vi "Kxx_Kxy_B_cs580.vi"() -> ()   [LabVIEW 2023]
uses:
  <instrlib>/Keithley 622x LV 2009/Keithley 622x.lvlib
  <instrlib>/Keithley 622x LV 2009/Utility/Typedefs/KE622x -- Instrument Type.ctl
  <vilib>/Analysis/NI_AALBase.lvlib
  <instrlib>/Keithley 24XX/Keithley 24XX.lvlib
  <vilib>/Analysis/1siggen.llb/Ramp Pattern by Samples.vi
  Global Variables/MQM Data Transfer All.vi
  <vilib>/Analysis/baseanly.llb/Mean (DBL).vi
  Typedefs/Kxx_Kxy_state_machine_cases.ctl
  Global Variables/Thermometers.vi
  <vilib>/Utility/file.llb/Read Delimited Spreadsheet (DBL).vi
  <vilib>/Instr/_visa.llb/VISA Configure Serial Port (Instr).vi
  <vilib>/Utility/file.llb/Write To Spreadsheet File (string).vi
panel:
  in  "Kxy data":dbl[](array[numeric])
  in  "Kxx data":dbl[](array[numeric])
  in  "T_avg data":dbl[](array[numeric])
  in  "dTxx":dbl
  in  "HTR Power":dbl
  in  "dTxy":dbl
  in  "T_avg":dbl
  in  "T_H Array":dbl[](array[numeric])
  in  "T_C1 Array":dbl[](array[numeric])
  in  "T_C2 Array":dbl[](array[numeric])
  in  "HTR Voltage Array":dbl[](array[numeric])
  in  "?":enum32{"Setup", "Plotting", "Error Readouts"}(tab)
  in  "DeltaT (fraction of tsp)":dbl=0.05
  in  "Sample_t":dbl
  in  "Sample_w":dbl
  in  "Sample_Lxx":dbl
  in  "Heater Current File (H, T, current)":path
  out "Heater Current \nArray":dbl[](array[numeric])
  out "Ramp Pattern":dbl[](array[numeric])
  in  "Tstart (K)":dbl=3.0
  in  "Tend (K)":dbl=4.0
  in  "Steps":i16=2
  in  "Log (on)\nLin (off) (Temperature setpoints)":bool=TRUE
  in  "Initial Heater Current (A)":dbl=1e-06
  in  "Hstart (Oe)":dbl
  in  "Hend (Oe)":dbl
  in  "Field Steps":i16=1
  in  "Log (on)\nLin (off)  (Field setpoints)":bool
  in  "Sample_Lxy":dbl=0.0005
  in  "Test?":bool
  in  "Calibration Only?":bool
  in  "Exchange gas?":bool
  in  "Preset Heater Current Array?":bool
  in  "T Current Source":refnum<visa-resource-name>="6221B"
  in  "HTR Current Source":refnum<visa-resource-name>="CS580-1"
  in  "DC Voltmeter":refnum<visa-resource-name>="2182"
  in  "Thermometer Frequency (Hz)":string="37"
  in  "Initial Thermometer Current (A)":string="1.4142e-7"
  in  "Final Field (Oe)":dbl
  in  "Final Temperature (K)":dbl=1.7
  in  "Filename":path=path "C:/User Data/Luke/Kxx/NaYSe2/NaYSe2_1p7_100K_log_100_9T_8_23_21"
  in  "Heater Only?":bool
  in  "Running avg size":dbl=500.0 format="%#_13g"
  in  "std/mean thresh":dbl=1e-05 format="%#_13g"
  in  "slope/mean thresh":dbl=1e-07 format="%#_13g"
  out "Kxx Plot":cluster{dbl[], dbl[]}(graph)
  out "Kxy Plot":cluster{dbl[], dbl[]}(graph)
  out "All Data":cluster{dbl[], dbl[]}[](graph)
  in  "Finish":bool
  out "Data Rate (ms)":u32
  in  "Delay (ms)":dbl=300.0
  in  "Quick Data Recording":bool=TRUE
  out "Tsp":dbl
  out "HTR_Current":dbl
  out "Mask":dbl
  out "HTR_Voltage":dbl
  out "T_H":dbl
  out "T_C1":dbl
  out "I_therm":dbl
  out "T_C2":dbl
  in  "Display Elements":cluster{"X":bool, "Y":bool, "Name":u16}[](array[cluster]) {"Name" items=["Time (ms)", "Temperature (K)", "Field (T)", "LI_1_X", "LI_1_theta", "LI_3_X", "LI_3_theta", "LI_2_X", "LI_2_theta", "DC_V", "DC_I", "mask", "tsp", "I_therm", "T_H", "T_C1", "T_C2", "Fieldsp"]}
  in  "X-Axis":u16(ring) items=["Linear", "Reciprocal", "Log10"]
  in  "Y-Axis":u16(ring) items=["Linear", "Reciprocal", "Log10"]
  out "Fieldsp":dbl
  out "Global Stop":bool
  out "Thermometers":cluster{"T_H":dbl, "T_C1":dbl, "T_C2":dbl}
  out "QD error out":errorcluster
  out "KE6221 error out":errorcluster
  out "KE2182 error out":errorcluster
  # "TURN ON HIGH VACUUM!"
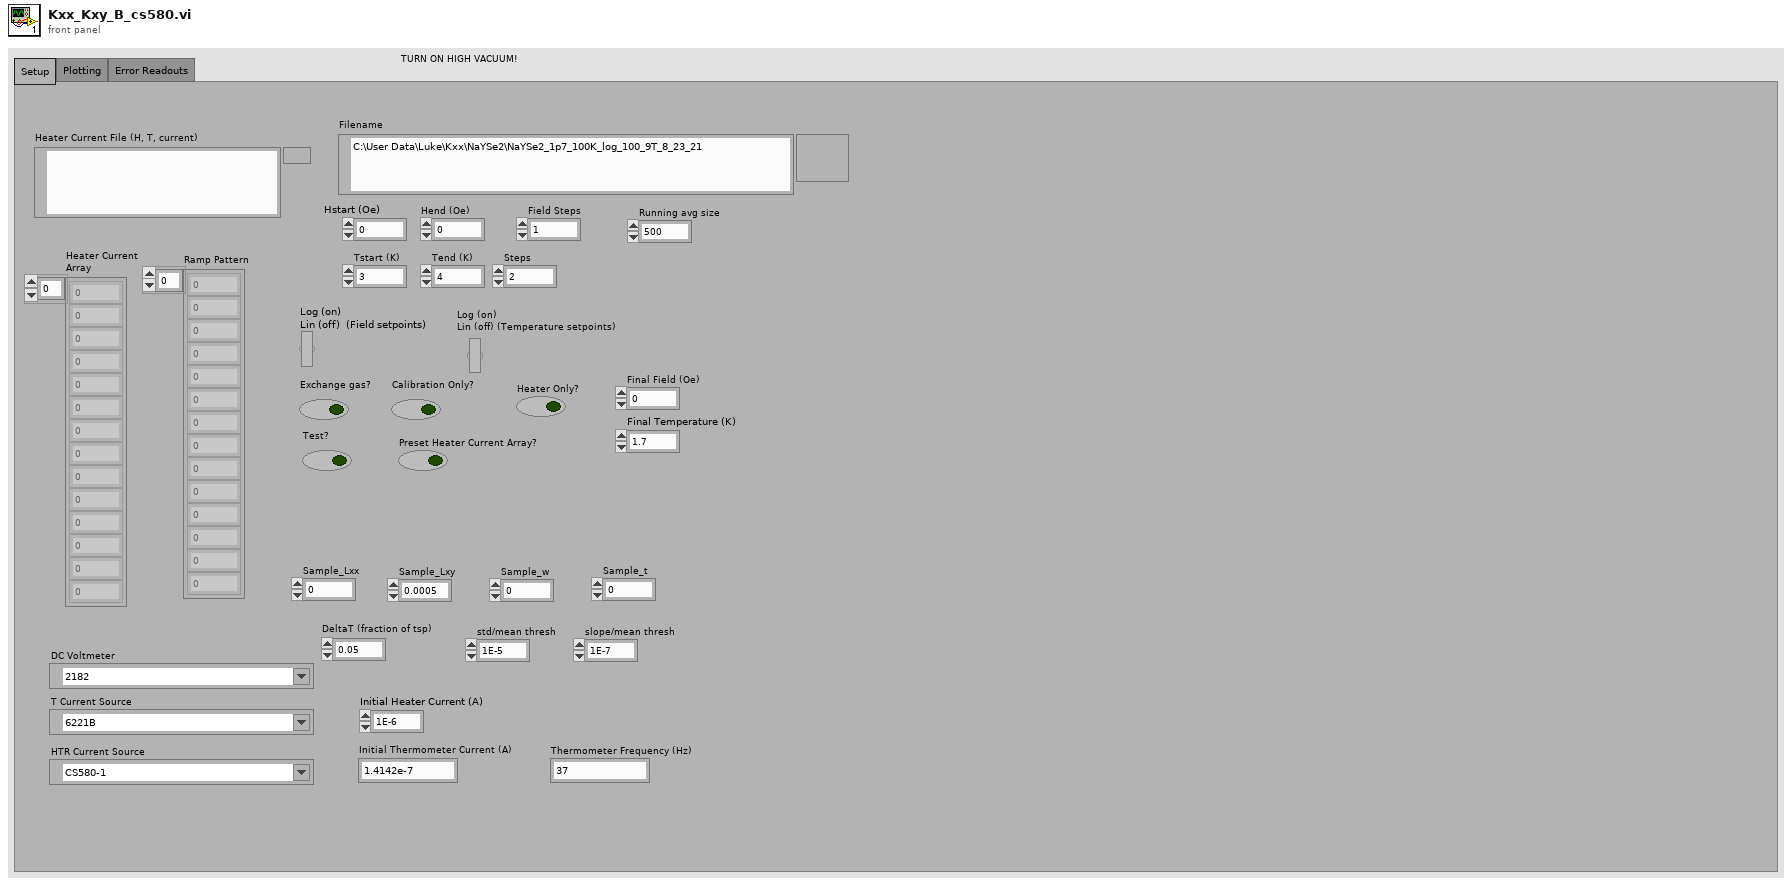
[diagram p1: front panel]
types:
  T1 = typedef "Keithley 622x.lvlib/KE622x -- Instrument Type.ctl" = enum16{"KE6220", "KE6221"}
  T2 = typedef "Kxx_Kxy_state_machine_cases.ctl" = enum16{"Initialize", "Wait to Stabilize (no heat)", "Measure (no heat)", "Turn on Heater, stabilize", "Measure (heat)", "Turn off Heater", "Assign Heater Current", "Plot Kxx, Kxy", "End"}
  T3 = cluster{"T_avg data":dbl[], "Kxx data":dbl[], "Kxy data":dbl[]}
  T4 = cluster{"T_avg":dbl, "dTxx":dbl, "dTxy":dbl, "HTR Power":dbl, "HTR Voltage Array":dbl[], "T_H Array":dbl[], "T_C1 Array":dbl[], "T_C2 Array":dbl[], "error out":errorcluster}
  T5 = typedef "ZI_Frontpanel_All.ctl" = cluster{"Lockin 1 Demod 0":cluster{"R(V)":dbl, "Theta (deg)":dbl, "Timestamp (ms)":u32, "X(V)":dbl, "Y(V)":dbl, "frequency (Hz)":dbl, "output voltage (V)":dbl}, "Lockin 2 Demod 0":cluster{"R(V)":dbl, "Theta (deg)":dbl, "Timestamp (ms)":u32, "X(V)":dbl, "Y(V)":dbl, "frequency (Hz)":dbl, "output voltage (V)":dbl}, "Lockin 3 Demod 0":cluster{"R(V)":dbl, "Theta (deg)":dbl, "Timestamp (ms)":u32, "X(V)":dbl, "Y(V)":dbl, "frequency (Hz)":dbl, "output voltage (V)":dbl}, "Lockin 4 Demod 0":cluster{"R(V)":dbl, "Theta (deg)":dbl, "Timestamp (ms)":u32, "X(V)":dbl, "Y(V)":dbl, "frequency (Hz)":dbl, "output voltage (V)":dbl}, "LI1 active":bool, "LI2 active":bool, "LI3 active":bool, "LI4 active":bool}
  T6 = typedef "PPMS_Status.ctl" = cluster{"Field":cluster{"Field (T)":dbl, "Field stable":bool, "Timestamp (ms)":u32}, "Temperature":cluster{"Temperature (K)":dbl, "Temperature stable":bool, "Timestamp (ms)":u32}}
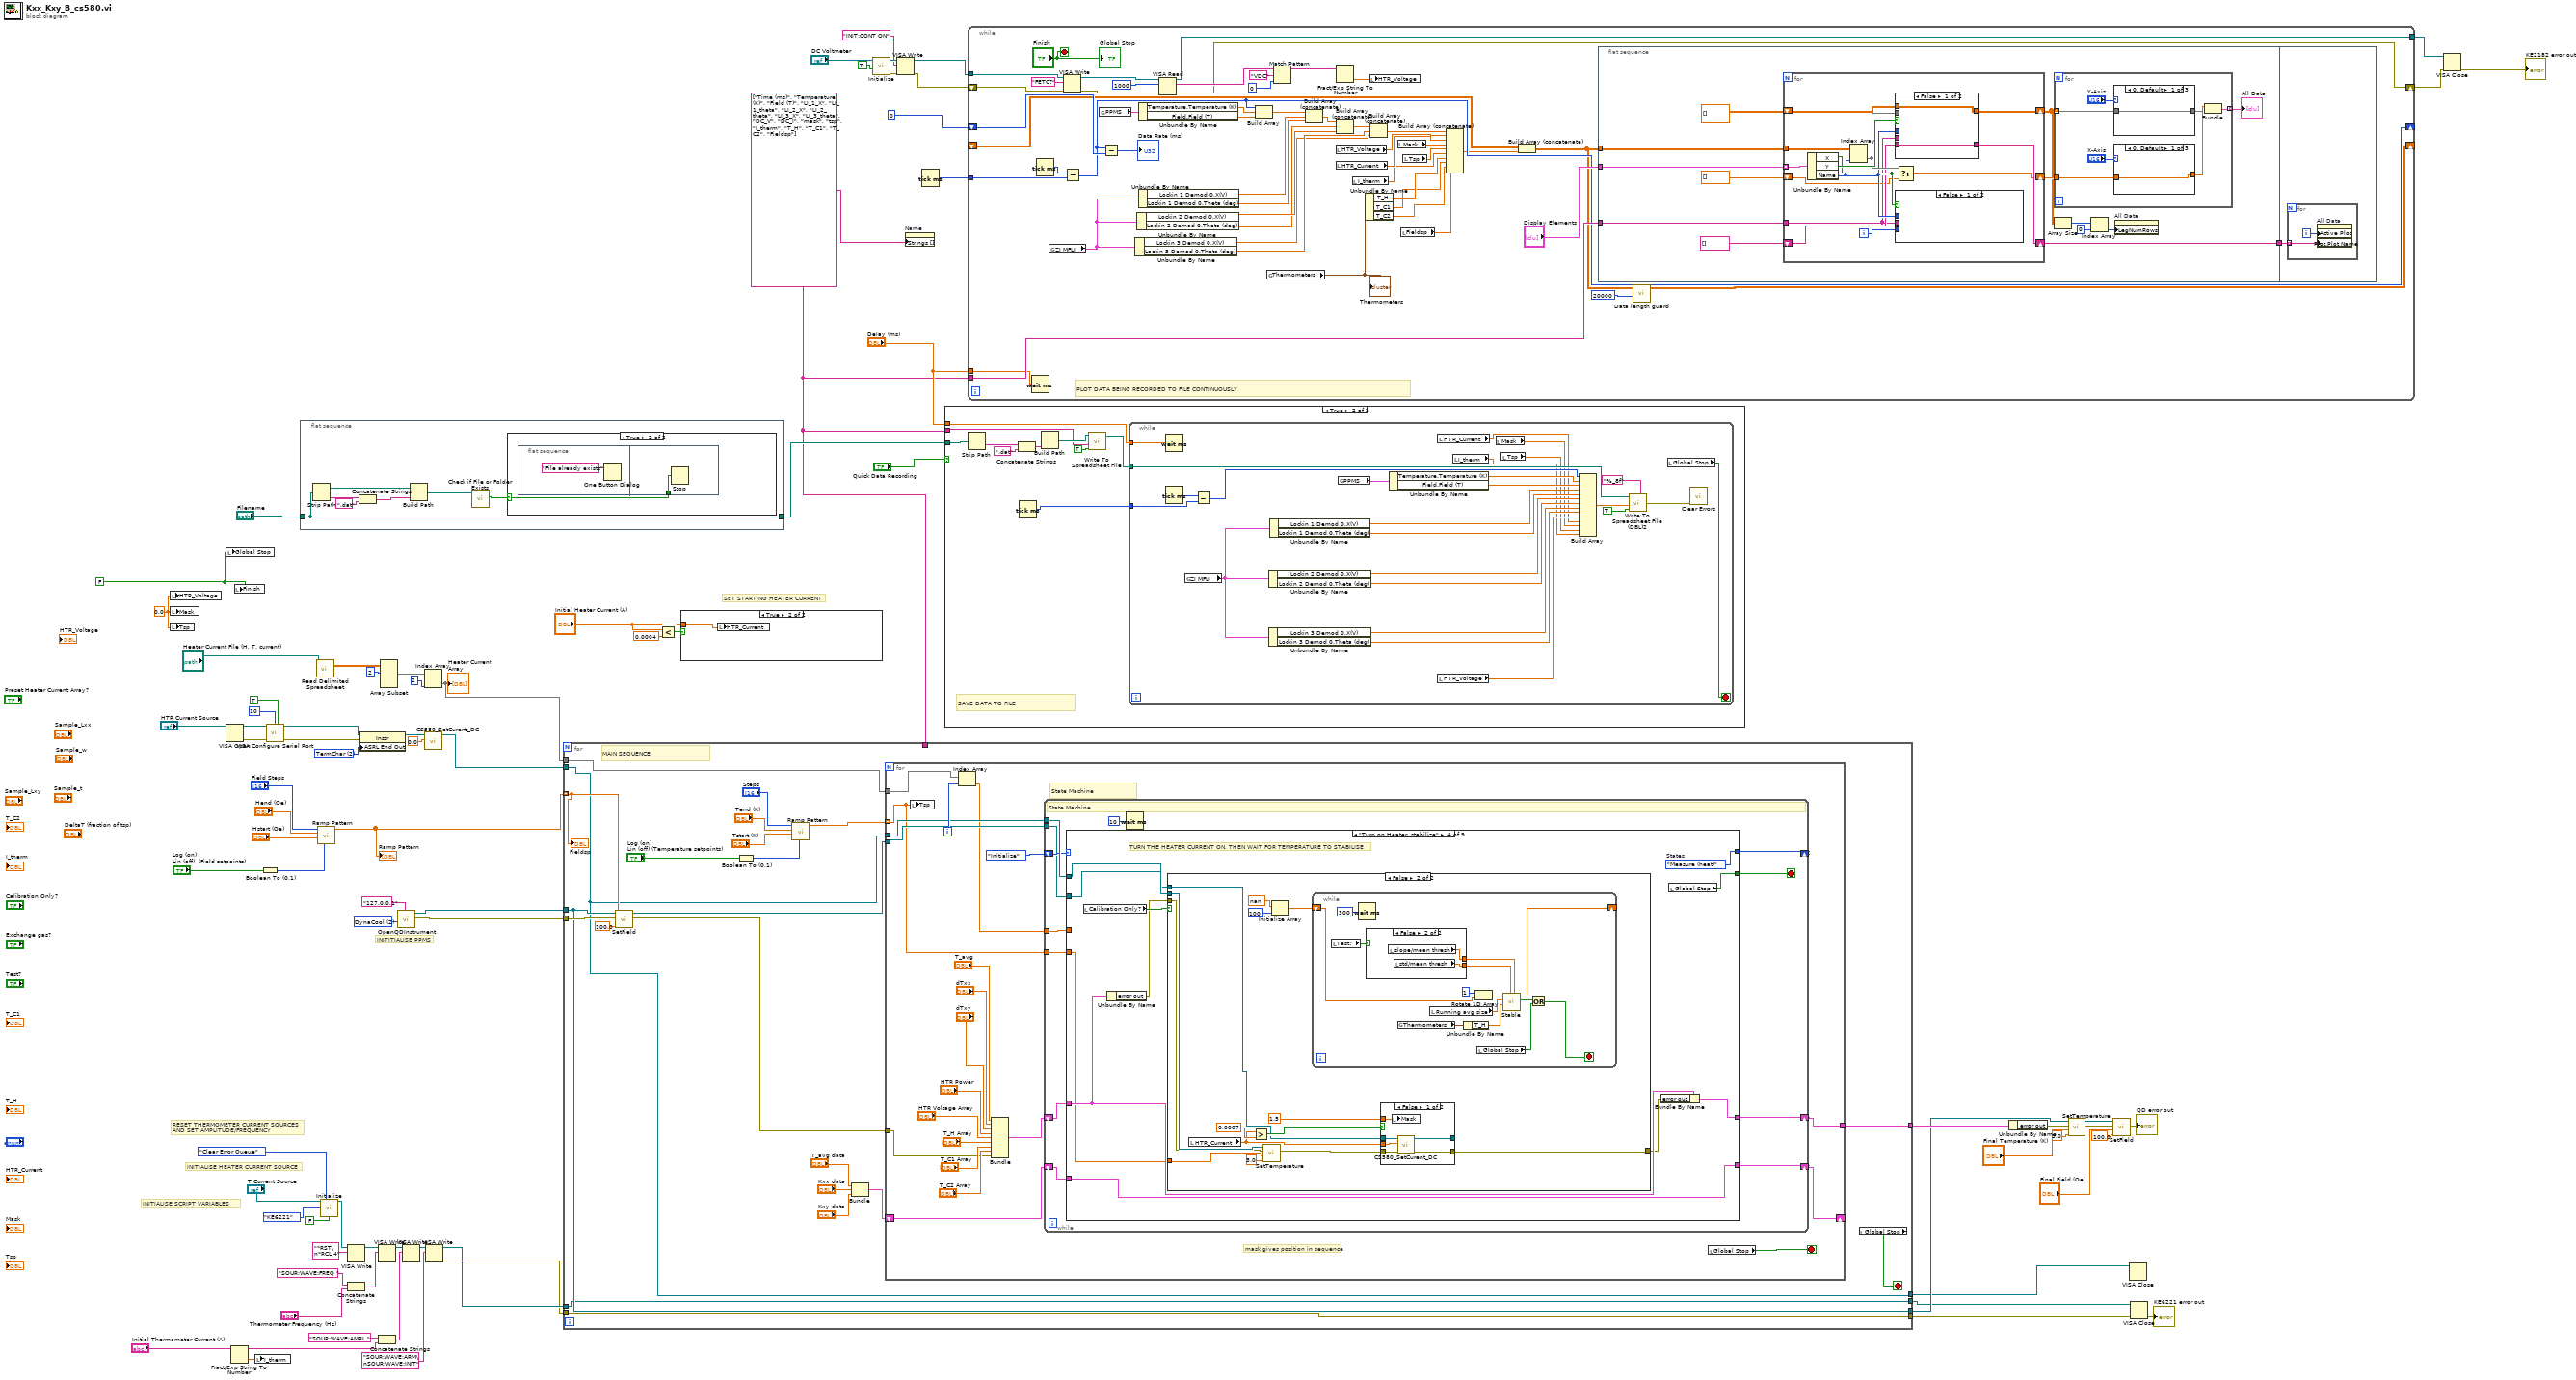
[diagram p0: block diagram]
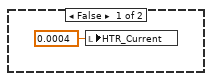
[diagram p2: hidden frame]
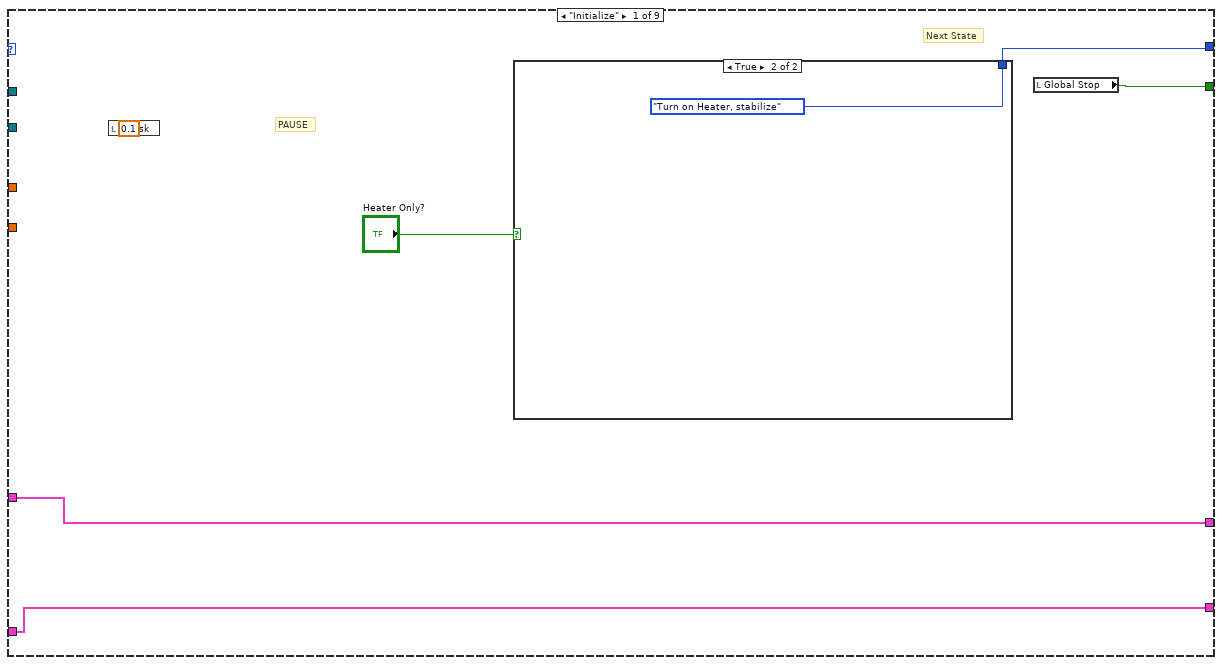
[diagram p4: hidden frame]
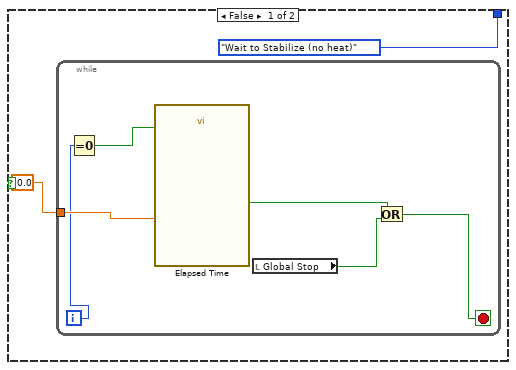
[diagram p5: hidden frame]
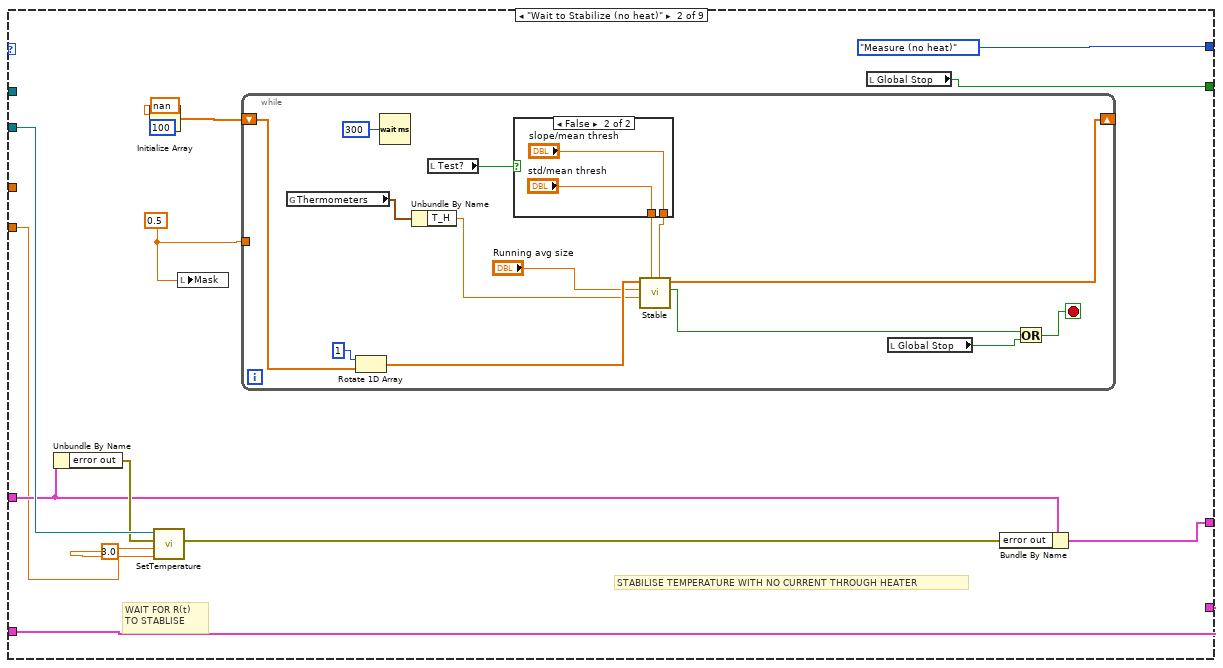
[diagram p6: hidden frame]
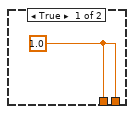
[diagram p7: hidden frame]
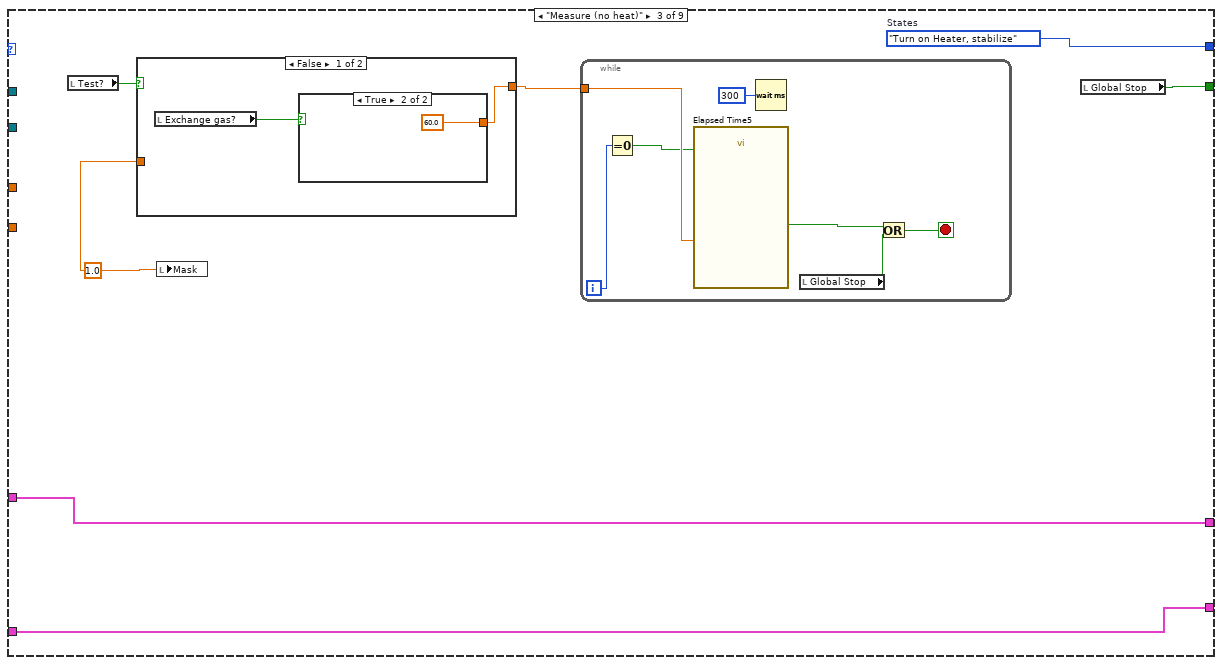
[diagram p8: hidden frame]
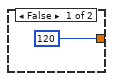
[diagram p9: hidden frame]
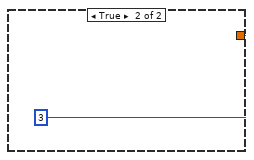
[diagram p10: hidden frame]
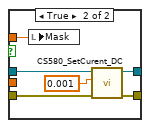
[diagram p12: hidden frame]
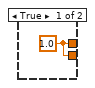
[diagram p13: hidden frame]
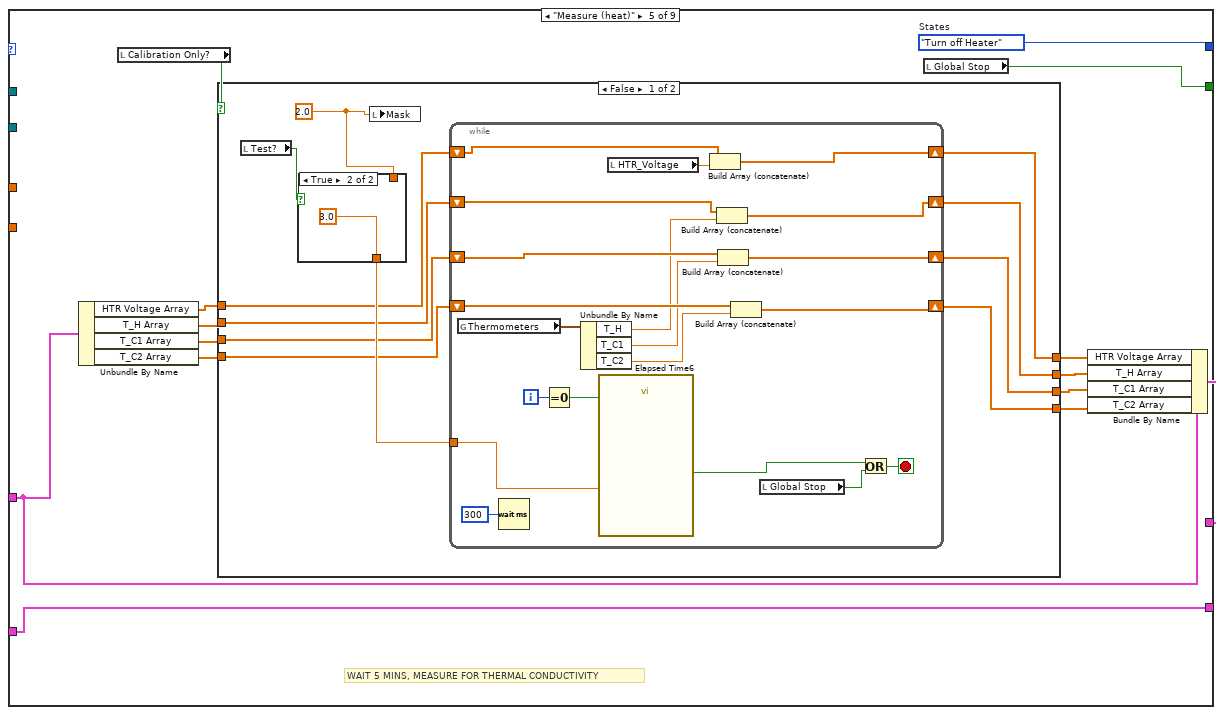
[diagram p14: hidden frame]
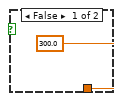
[diagram p15: hidden frame]
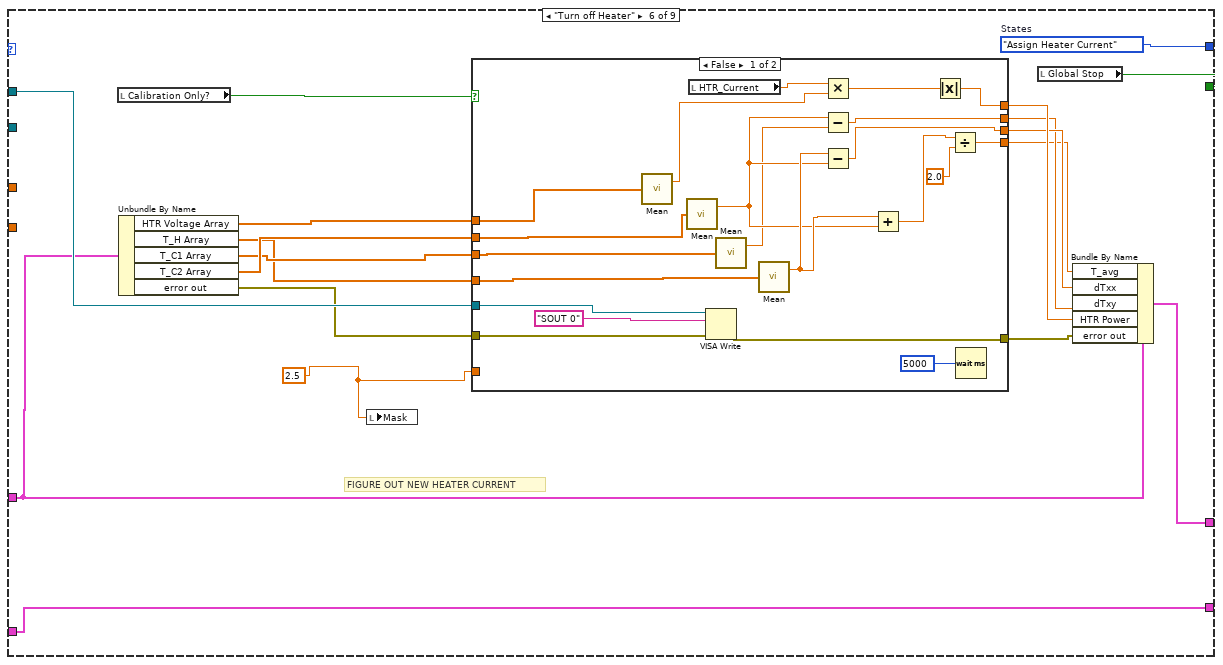
[diagram p17: hidden frame]
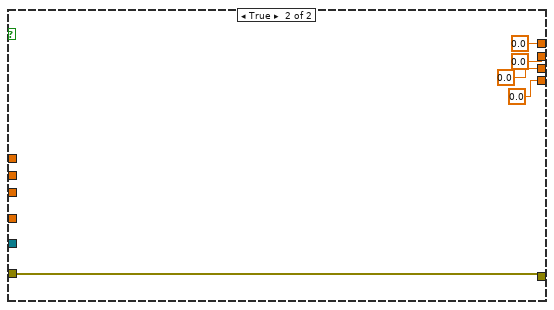
[diagram p18: hidden frame]
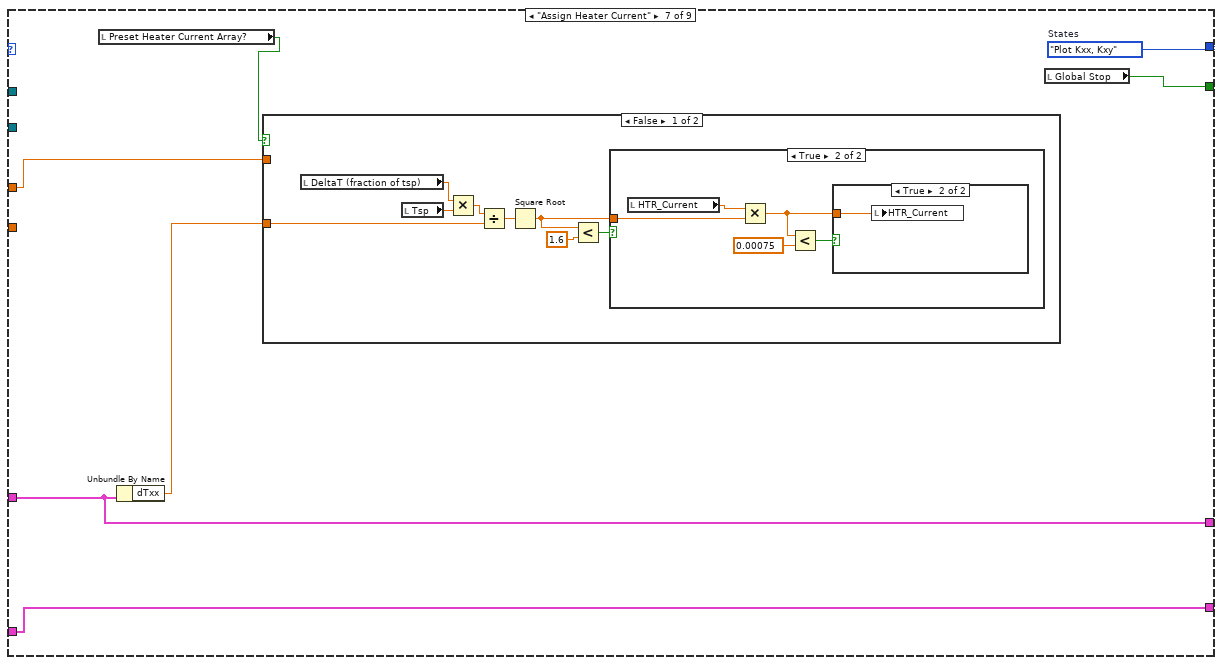
[diagram p19: hidden frame]
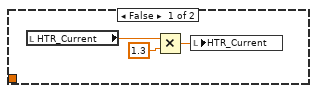
[diagram p20: hidden frame]
diagram:
  w2 = FALSE ("Calibration confirmed")
  w1 = string[] ["Time (ms)", "Temperature (K)", "Field (T)", "LI_1_X", "LI_1_theta", "LI_2_X", "LI_2_theta", "LI_3_X", "LI_3_theta", "DC_V", "DC_I", "mask", "tsp", "I_therm", "T_H", "T_C1", "T_C2", "Fieldsp"] ("element")
  w53 = u16 2 items=["None", "Last Bit", "TermChar", "Break"] ("Serial Settings:End Mode for Writes")
  w71 = 0.0 ("Mask")
  w78 = 2 items=["PPMS", "VersaLab", "DynaCool", "SVSM"] ("Instrument Type")
  # "SET STARTING HEATER CURRENT"
  # "INITIALISE HEATER CURRENT SOURCE"
  # "RESET THERMOMETER CURRENT SOURCES\nAND SET AMPLITUDE/FREQUENCY"
  # "INITITIALISE PPMS"
  # "INITIALISE SCRIPT VARIABLES"
  n1 = local write "HTR_Voltage"(w71) -> ()
  n2 = local write "Mask"(w71) -> ()
  n3 = local write "Tsp"(w71) -> ()
  n4 = VISA Open(VISA resource name="HTR Current Source") -> (VISA resource name=w49:refnum<visa-resource-name>, error out=w50:errorcluster)  [unwired: 4 in]
  n5 = local write "Global Stop"(w2) -> ()
  n6 = Fract/Exp String To Number(string="Initial Thermometer Current (A)") -> (number=w61:dbl)  [unwired: 3 in, 1 out]
  n7 = local write "Finish"(w2) -> ()
  n8 = local write "I_therm"(w61) -> ()
  n9 = Boolean To (0,1)(Boolean="Log (on)\nLin (off)  (Field setpoints)") -> (0, 1=w56:i16)
  n10 = call-poly "VISA Configure Serial Port"("VISA resource name"=w49, "termination char\n(0xA = '\\n' = LF)"=u8 10 ("termination char\n(0xA = '\\n' = LF)"), "Enable Termination\nChar (T)"=TRUE ("Enable Termination\nChar (T)"), "error in (no error)"=w50) -> ("VISA resource name out"=w51:refnum<visa-resource-name>, "error out"=w52:errorcluster)  [unwired: 10 in]
  n11 = flat-sequence {
    tunnel: "Filename" -> [w85]
    tunnel: [w85] -> w22
    frame #0 {
      n12 = Strip Path(path=w85) -> (stripped path=w89:path, name=w86:string)
      n13 = Concatenate Strings(w86, ".dat") -> (w88:string)
      n14 = Build Path(base path=w89, name or relative path=w88) -> (appended path=w84:path)
      n15 = call <vilib>:"Check if File or Folder Exists.vi"("path"=w84) -> ("file or folder exists?"=w83:bool)  [unwired: 8 in, 2 out]
      n16 = case shown="True" w83 {
        selector: w83 -> [_ w90]
        frame False {
        }
        frame True {
          n17 = flat-sequence {
            tunnel: w90 -> [w92]
            frame #0 {
              n18 = One Button Dialog(message="File already exists") -> ()  [unwired: 1 in, 1 out]
            }
            frame #1 {
              n19 = Stop(stop? (T)=w92) -> ()
            }
          }
        }
      }
    }
  }
  n20 = call-poly <vilib>:"Read Delimited Spreadsheet.vi"("file path (dialog if empty)"="Heater Current File (H, T, current)") -> ("all rows"=w44:dbl[][])  [unwired: 9 in, 5 out]
  n21 = call-poly <vilib>:"Ramp Pattern.vi"("type"=w56, "start"="Hstart (Oe)", "end"="Hend (Oe)", "samples"="Field Steps") -> ("Ramp Pattern"=w38:dbl[])  [unwired: 6 in, 1 out]
  "Ramp Pattern" <- w38
  n22 = call <instrlib>:"Initialize.vi"("VISA resource name"="T Current Source", "Error Queue Option"=enum16{"Clear Error Queue", "Error Query"}."Clear Error Queue", "Instrument Type"=KE622x_--_Instrument_Type."KE6221", "Reset? (T)"=FALSE) -> ("VISA resource name out"=w69:refnum<visa-resource-name>)  [unwired: 10 in, 1 out]
  n23 = VISA Write(VISA resource name=w69, write buffer="*RST\n*RCL 4") -> (VISA resource name out=w63:refnum<visa-resource-name>)  [unwired: 1 in, 2 out]
  n24 = Concatenate Strings("SOUR:WAVE:FREQ " ("string"), "Thermometer Frequency (Hz)") -> (w68:string)
  n25 = property class="Instr"(reference=w51, error in=w52, "ASRL End Out"=w53) -> (reference out=w47:refnum<visa-resource-name>)  [unwired: 1 out]
  n26 = VISA Write(VISA resource name=w63, write buffer=w68) -> (VISA resource name out=w62:refnum<visa-resource-name>)  [unwired: 1 in, 2 out]
  n27 = Concatenate Strings("SOUR:WAVE:AMPL " ("string"), "Initial Thermometer Current (A)") -> (w65:string)
  n28 = Array Subset(array=w44, index (row)=2 ("index")) -> (w42:dbl[][])  [unwired: 3 in]
  n29 = call <instrlib>:"OpenQDInstrument.vi"("IP Address"="127.0.0.1", "Instrument Type"=w78) -> ("error out"=w21:errorcluster, "Instrument Ref"=w19:refnum<k24>)  [unwired: 6 in]
  n30 = VISA Write(VISA resource name=w62, write buffer=w65) -> (VISA resource name out=w39:refnum<visa-resource-name>)  [unwired: 1 in, 2 out]
  n31 = Index Array(array=w42, index (col)=2 ("disabled index (col)")) -> (element=w37:dbl[])  [unwired: 1 in]
  "Heater Current \nArray" <- w37
  n32 = call "CS580_SetCurent_DC.vi"("Current (A)"=0.0, "VISA Refnum in"=w47) -> ("VISA resource name out"=w20:refnum<visa-resource-name>)  [unwired: 8 in, 1 out]
  n33 = VISA Write(VISA resource name=w39, write buffer="SOUR:WAVE:ARM\nSOUR:WAVE:INIT") -> (VISA resource name out=w12:refnum<visa-resource-name>, error out=w8:errorcluster)  [unwired: 1 in, 1 out]
  n34 = for {
    tunnel: w38 -> [w114] mode=indexing
    tunnel: w19 -> [w97]
    tunnel: w21 -> [w112]
    tunnel: w37 -> [w105]
    tunnel: w20 -> [w93]
    tunnel: [w98] -> w14
    tunnel: w12 -> [w96]
    tunnel: [w97] -> w11
    tunnel: [w96] -> w10
    tunnel: w8 -> [w95]
    tunnel: [w95] -> w7
    tunnel: [w93] -> w3
    tunnel: w1 -> [_]
    stop <- w94 stop-if-true
    # "MAIN SEQUENCE"
    n35 = call <instrlib>:"SetField.vi"("Rate"=100.0, "Field"=w114, "error in (no error)"=w112, "Instrument Ref In"=w97) -> ("error out"=w104:errorcluster, "Instrument Ref Out"=w103:refnum<k24>)  [unwired: 3 in, 1 out]
    n36 = Boolean To (0,1)(Boolean="Log (on)\nLin (off) (Temperature setpoints)") -> (0, 1=w109:i16)
    n37 = call-poly <vilib>:"Ramp Pattern.vi"("type"=w109, "start"="Tstart (K)", "end"="Tend (K)", "samples"="Steps") -> ("Ramp Pattern"=w111:dbl[])  [unwired: 6 in, 1 out]
    n38 = Bundle("T_avg data"="T_avg data", "Kxx data"="Kxx data", "Kxy data"="Kxy data") -> (w99:T3)  [unwired: 1 in]
    n39 = for {
      tunnel: w111 -> [w117] mode=indexing
      tunnel: w105 -> [w135]
      tunnel: w104 -> [w122]
      tunnel: w93 -> [w132]
      tunnel: w103 -> [w131]
      shift-right: [w116] -> _
      shift-left: w99 -> [w115]
      tunnel: [w119] -> w98
      i -> [w134]
      stop <- w118 stop-if-true
      # "State Machine"
      # "mask gives position in sequence"
      n40 = local write "Tsp"(w117) -> ()
      n41 = Index Array(array=w135, index=w134) -> (element=w120:dbl)
      n42 = Bundle("T_avg"="T_avg", "dTxx"="dTxx", "dTxy"="dTxy", "HTR Power"="HTR Power", "HTR Voltage Array"="HTR Voltage Array", "T_H Array"="T_H Array", "T_C1 Array"="T_C1 Array", "T_C2 Array"="T_C2 Array", "error out"=w122) -> (w121:T4)  [unwired: 1 in]
      n43 = while {
        shift-right: [w147] -> _
        shift-left: Kxx_Kxy_state_machine_cases."Initialize" -> [w144]
        tunnel: w132 -> [w145]
        tunnel: w131 -> [w140]
        shift-right: [w143] -> w119
        shift-left: w121 -> [w142]
        tunnel: w120 -> [w141]
        tunnel: w117 -> [w138]
        shift-right: [w137] -> w116
        shift-left: w115 -> [w136]
        stop <- w139 stop-if-true
        # "State Machine"
        n44 = case shown="\"Turn on Heater, stabilize\"" w144 {
          selector: w144 -> [_ _ _ _ _ _ _ _ w418]
          tunnel: w140 -> [_ w172 _ w222 _ _ _ _ _]
          tunnel: [w152 Kxx_Kxy_state_machine_cases."Measure (no heat)" w198 w220 w280 w334 w368 w406 w418] -> w147
          tunnel: w145 -> [_ _ _ w221 _ w335 _ _ _]
          tunnel: [w151 w168 w197 w216 w271 w322 w366 w405 w417] -> w143
          tunnel: w142 -> [w151 w169 w197 w218 w270 w329 w366 w405 w417]
          tunnel: w136 -> [w150 w167 w196 w215 w269 w321 w365 w396 w416]
          tunnel: [w150 w167 w196 w215 w269 w321 w365 w392 w416] -> w137
          tunnel: w141 -> [_ _ _ _ _ _ w364 _ _]
          tunnel: [w149 w166 w195 w214 w268 w320 w363 w389 TRUE] -> w139
          tunnel: w138 -> [_ w165 _ w213 _ _ _ _ _]
          frame "Initialize" {
            # "Next State"
            # "PAUSE"
            n45 = local write "Mask"(0.1 ("Mask")) -> ()
            n46 = case shown="True" "Heater Only?" {
              tunnel: [Kxx_Kxy_state_machine_cases."Wait to Stabilize (no heat)" Kxx_Kxy_state_machine_cases."Turn on Heater, stabilize"] -> w152
              frame False {
                n47 = while {
                  tunnel: 10.0 ("Time Target (s)") -> [w161]
                  i -> [w157]
                  stop <- w158 stop-if-true
                  n48 = Equal To 0?(x=w157) -> (x = 0?=w156:bool)
                  n49 = call "Elapsed Time"("Time Target (s)"=w161, "Reset"=w156) -> ("Time has Elapsed"=w160:bool)  [unwired: 10 in, 7 out]
                  n50 = local read "Global Stop"() -> (w159:bool)
                  n51 = Or(x=w160, y=w159) -> (x .or. y?=w158:bool)
                }
              }
              frame True {
              }
            }
            n52 = local read "Global Stop"() -> (w149:bool)
          }
          frame "Wait to Stabilize (no heat)" {
            w163 = 0.5 ("Mask")
            # "STABILISE TEMPERATURE WITH NO CURRENT THROUGH HEATER"
            # "WAIT FOR R(t)\nTO STABLISE"
            n53 = Unbundle By Name(w169) -> ("error out"=w170:errorcluster)
            n54 = Initialize Array(nan ("Element"), 100) -> (w176:dbl[])
            n55 = call <instrlib>:"SetTemperature.vi"("Rate"=3.0, "Temperature"=w165, "error in (no error)"=w170, "Instrument Ref In"=w172) -> ("error out"=w164:errorcluster)  [unwired: 3 in, 2 out]
            n56 = local write "Mask"(w163) -> ()
            n57 = while {
              shift-right: [w179] -> _
              shift-left: w176 -> [w189]
              tunnel: w163 -> [_]
              stop <- w185 stop-if-true
              n58 = global read "Thermometers.vi" "Thermometers"() -> (w184:cluster{"T_H":dbl, "T_C1":dbl, "T_C2":dbl})
              n59 = Rotate 1D Array(1:w189, 2:1 ("n")) -> (0:w183:dbl[])
              n60 = Wait (ms)(milliseconds to wait=u32 300) -> ()  [unwired: 1 out]
              n61 = Unbundle By Name(w184) -> ("T_H"=w181:dbl)
              n62 = local read "Test?"() -> (w187:bool)
              n63 = case shown="False" w187 {
                tunnel: [w191 "slope/mean thresh"] -> w180
                tunnel: [w191 "std/mean thresh"] -> w177
                frame True {
                  w191 = 1.0 ("y")
                }
                frame False {
                }
              }
              n64 = call "Stable.vi"("slope/mean thresh"=w180, "std/mean thresh"=w177, "New data point"=w181, "Number of points"="Running avg size", "Array in"=w183) -> ("Stable?"=w178:bool, "Array out"=w179:dbl[])  [unwired: 5 in]
              n65 = local read "Global Stop"() -> (w186:bool)
              n66 = Or(x=w178, y=w186) -> (x .or. y?=w185:bool)
            }
            n67 = local read "Global Stop"() -> (w166:bool)
            n68 = Bundle By Name(cluster=w169, "error out"=w164) -> (w168:T4)
          }
          frame "Measure (no heat)" {
            w198 = Kxx_Kxy_state_machine_cases."Turn on Heater, stabilize"  # States
            w194 = 1.0 ("Mask")
            n69 = local read "Test?"() -> (w200:bool)
            n70 = case shown="False" w200 {
              tunnel: [w201 u32 3 ("milliseconds to wait")] -> w199
              tunnel: w194 -> [_ _]
              frame False {
                n71 = local read "Exchange gas?"() -> (w202:bool)
                n72 = case shown="True" w202 {
                  tunnel: [120 60.0 ("Time to Wait (s)")] -> w201
                  frame False {
                  }
                  frame True {
                  }
                }
              }
              frame True {
              }
            }
            n73 = local write "Mask"(w194) -> ()
            n74 = while {
              tunnel: w199 -> [w210]
              i -> [w207]
              stop <- w209 stop-if-true
              n75 = Equal To 0?(x=w207) -> (x = 0?=w206:bool)
              n76 = call "Elapsed Time5"("Time Target (s)"=w210, "Reset"=w206) -> ("Time has Elapsed"=w208:bool)  [unwired: 10 in, 7 out]
              n77 = Wait (ms)(milliseconds to wait=u32 300) -> ()  [unwired: 1 out]
              n78 = local read "Global Stop"() -> (w212:bool)
              n79 = Or(x=w208, y=w212) -> (x .or. y?=w209:bool)
            }
            n80 = local read "Global Stop"() -> (w195:bool)
          }
          frame "Turn on Heater, stabilize" {
            w220 = Kxx_Kxy_state_machine_cases."Measure (heat)"  # States
            # "TURN THE HEATER CURRENT ON, THEN WAIT FOR TEMPERATURE TO STABILISE"
            n81 = local read "Calibration Only?"() -> (w223:bool)
            n82 = Unbundle By Name(w218) -> ("error out"=w219:errorcluster)
            n83 = case shown="False" w223 {
              tunnel: w222 -> [_ w238]
              tunnel: w219 -> [w224 w230]
              tunnel: [w224 w231] -> w217
              tunnel: w221 -> [_ w232]
              tunnel: w213 -> [_ w227]
              frame True {
              }
              frame False {
                n84 = local read "HTR_Current"() -> (w225:dbl)
                n85 = Greater?(x=w225, y=0.0007) -> (0:w233:bool)
                n86 = call <instrlib>:"SetTemperature.vi"("Rate"=3.0, "Temperature"=w227, "error in (no error)"=w230, "Instrument Ref In"=w238) -> ("error out"=w229:errorcluster)  [unwired: 3 in, 2 out]
                n87 = Initialize Array(nan ("Element"), 100) -> (w237:dbl[])
                n88 = while {
                  shift-right: [w261] -> _
                  shift-left: w237 -> [w263]
                  stop <- w259 stop-if-true
                  n89 = local read "Test?"() -> (w260:bool)
                  n90 = Wait (ms)(milliseconds to wait=u32 300) -> ()  [unwired: 1 out]
                  n91 = case shown="False" w260 {
                    tunnel: [w265 w267] -> w253
                    tunnel: [w265 w266] -> w252
                    frame True {
                      w265 = 1.0 ("y")
                    }
                    frame False {
                      n92 = local read "slope/mean thresh"() -> (w267:dbl)
                      n93 = local read "std/mean thresh"() -> (w266:dbl)
                    }
                  }
                  n94 = global read "Thermometers.vi" "Thermometers"() -> (w257:cluster{"T_H":dbl, "T_C1":dbl, "T_C2":dbl})
                  n95 = local read "Running avg size"() -> (w251:dbl)
                  n96 = Unbundle By Name(w257) -> ("T_H"=w254:dbl)
                  n97 = Rotate 1D Array(1:w263, 2:1 ("n")) -> (0:w255:dbl[])
                  n98 = local read "Global Stop"() -> (w258:bool)
                  n99 = call "Stable.vi"("slope/mean thresh"=w253, "std/mean thresh"=w252, "New data point"=w254, "Number of points"=w251, "Array in"=w255) -> ("Stable?"=w256:bool, "Array out"=w261:dbl[])  [unwired: 5 in]
                  n100 = Or(x=w256, y=w258) -> (x .or. y?=w259:bool)
                }
                n101 = case shown="False" w233 {
                  tunnel: w229 -> [w242 w250]
                  tunnel: w232 -> [w243 w249]
                  tunnel: [w240 w248] -> w231
                  tunnel: [w241 w247] -> _
                  tunnel: w225 -> [w244 _]
                  tunnel: 1.5 ("Mask") -> [w239 w245]
                  frame False {
                    n102 = local write "Mask"(w239) -> ()
                    n103 = call "CS580_SetCurent_DC.vi"("error in"=w242, "Current (A)"=w244, "VISA Refnum in"=w243) -> ("error out"=w240:errorcluster, "VISA resource name out"=w241:refnum<visa-resource-name>)  [unwired: 7 in]
                  }
                  frame True {
                    n104 = local write "Mask"(w245) -> ()
                    n105 = call "CS580_SetCurent_DC.vi"("error in"=w250, "Current (A)"=0.001, "VISA Refnum in"=w249) -> ("error out"=w248:errorcluster, "VISA resource name out"=w247:refnum<visa-resource-name>)  [unwired: 7 in]
                  }
                }
              }
            }
            n106 = Bundle By Name(cluster=w218, "error out"=w217) -> (w216:T4)
            n107 = local read "Global Stop"() -> (w214:bool)
          }
          frame "Measure (heat)" {
            w280 = Kxx_Kxy_state_machine_cases."Turn off Heater"  # States
            # "WAIT 5 MINS, MEASURE FOR THERMAL CONDUCTIVITY"
            n108 = Unbundle By Name(w270) -> ("HTR Voltage Array"=w279:dbl[], "T_H Array"=w278:dbl[], "T_C1 Array"=w277:dbl[], "T_C2 Array"=w276:dbl[])
            n109 = local read "Calibration Only?"() -> (w281:bool)
            n110 = case shown="False" w281 {
              tunnel: w279 -> [w290 w318]
              tunnel: w278 -> [w287 w317]
              tunnel: w277 -> [w286 w316]
              tunnel: w276 -> [w285 w315]
              tunnel: [w289 w318] -> w275
              tunnel: [w284 w317] -> w274
              tunnel: [w283 w316] -> w273
              tunnel: [w282 w315] -> w272
              frame False {
                w288 = 2.0 ("Mask")
                n111 = local read "Test?"() -> (w292:bool)
                n112 = case shown="True" w292 {
                  tunnel: [300.0 3.0] -> w291
                  tunnel: w288 -> [_ _]
                  frame False {
                  }
                  frame True {
                  }
                }
                n113 = local write "Mask"(w288) -> ()
                n114 = while {
                  shift-right: [w313] -> w284
                  shift-left: w287 -> [w314]
                  shift-right: [w311] -> w282
                  shift-left: w285 -> [w312]
                  shift-right: [w309] -> w289
                  shift-left: w290 -> [w310]
                  shift-right: [w303] -> w283
                  shift-left: w286 -> [w304]
                  tunnel: w291 -> [w299]
                  i -> [w306]
                  stop <- w300 stop-if-true
                  n115 = global read "Thermometers.vi" "Thermometers"() -> (w298:cluster{"T_H":dbl, "T_C1":dbl, "T_C2":dbl})
                  n116 = Wait (ms)(milliseconds to wait=u32 300) -> ()  [unwired: 1 out]
                  n117 = Equal To 0?(x=w306) -> (x = 0?=w305:bool)
                  n118 = Unbundle By Name(w298) -> ("T_H"=w297:dbl, "T_C1"=w296:dbl, "T_C2"=w295:dbl)
                  n119 = call "Elapsed Time6"("Time Target (s)"=w299, "Reset"=w305) -> ("Time has Elapsed"=w302:bool)  [unwired: 10 in, 7 out]
                  n120 = local read "HTR_Voltage"() -> (w308:dbl)
                  n121 = Build Array (concatenate)(w310, w308) -> (w309:dbl[])
                  n122 = Build Array (concatenate)(w314, w297) -> (w313:dbl[])
                  n123 = Build Array (concatenate)(w304, w296) -> (w303:dbl[])
                  n124 = Build Array (concatenate)(w312, w295) -> (w311:dbl[])
                  n125 = local read "Global Stop"() -> (w301:bool)
                  n126 = Or(x=w302, y=w301) -> (x .or. y?=w300:bool)
                }
              }
              frame True {
              }
            }
            n127 = local read "Global Stop"() -> (w268:bool)
            n128 = Bundle By Name(cluster=w270, "HTR Voltage Array"=w275, "T_H Array"=w274, "T_C1 Array"=w273, "T_C2 Array"=w272) -> (w271:T4)
          }
          frame "Turn off Heater" {
            w319 = 2.5 ("Mask")
            w334 = Kxx_Kxy_state_machine_cases."Assign Heater Current"  # States
            # "FIGURE OUT NEW HEATER CURRENT"
            n129 = local read "Calibration Only?"() -> (w336:bool)
            n130 = Unbundle By Name(w329) -> ("HTR Voltage Array"=w333:dbl[], "T_H Array"=w330:dbl[], "T_C1 Array"=w331:dbl[], "T_C2 Array"=w332:dbl[], "error out"=w328:errorcluster)
            n131 = local write "Mask"(w319) -> ()
            n132 = case shown="False" w336 {
              tunnel: w335 -> [w349 _]
              tunnel: w328 -> [w348 w362]
              tunnel: w332 -> [w338 _]
              tunnel: w330 -> [w339 _]
              tunnel: w333 -> [w340 _]
              tunnel: [w356 0.0] -> w325
              tunnel: [w341 0.0] -> w326
              tunnel: [w350 0.0] -> w323
              tunnel: [w347 w362] -> w327
              tunnel: w331 -> [w337 _]
              tunnel: [w343 0.0] -> w324
              tunnel: w319 -> [_ _]
              frame False {
                n133 = call-poly <vilib>:"Mean.vi"("X"=w340) -> ("mean"=w354:dbl)  [unwired: 1 out]
                n134 = call-poly <vilib>:"Mean.vi"("X"=w338) -> ("mean"=w345:dbl)  [unwired: 1 out]
                n135 = local read "HTR_Current"() -> (w355:dbl)
                n136 = VISA Write(VISA resource name=w349, write buffer="SOUT 0", error in (no error)=w348) -> (error out=w347:errorcluster)  [unwired: 2 out]
                n137 = call-poly <vilib>:"Mean.vi"("X"=w337) -> ("mean"=w344:dbl)  [unwired: 1 out]
                n138 = call-poly <vilib>:"Mean.vi"("X"=w339) -> ("mean"=w353:dbl)  [unwired: 1 out]
                n139 = Multiply(x=w355, y=w354) -> (x*y=w342:dbl)
                n140 = Subtract(x=w345, y=w344) -> (x-y=w343:dbl)
                n141 = Subtract(x=w353, y=w345) -> (x-y=w356:dbl)
                n142 = Add(x=w353, y=w345) -> (x+y=w352:dbl)
                n143 = Absolute Value(x=w342) -> (abs(x)=w341:dbl)
                n144 = Divide(x=w352, y=2.0) -> (x/y=w350:dbl)
                n145 = Wait (ms)(milliseconds to wait=u32 5000) -> ()  [unwired: 1 out]
              }
              frame True {
              }
            }
            n146 = local read "Global Stop"() -> (w320:bool)
            n147 = Bundle By Name(cluster=w329, "T_avg"=w323, "dTxx"=w325, "dTxy"=w324, "HTR Power"=w326, "error out"=w327) -> (w322:T4)
          }
          frame "Assign Heater Current" {
            w368 = Kxx_Kxy_state_machine_cases."Plot Kxx, Kxy"  # States
            n148 = local read "Preset Heater Current Array?"() -> (w369:bool)
            n149 = Unbundle By Name(w366) -> ("dTxx"=w367:dbl)
            n150 = case shown="False" w369 {
              tunnel: w367 -> [w375 _]
              tunnel: w364 -> [_ w388]
              frame False {
                n151 = local read "DeltaT (fraction of tsp)"() -> (w370:dbl)
                n152 = local read "Tsp"() -> (w377:dbl)
                n153 = Multiply(x=w370, y=w377) -> (x*y=w376:dbl)
                n154 = Divide(x=w376, y=w375) -> (x/y=w374:dbl)
                n155 = Square Root(x=w374) -> (sqrt(x)=w373:dbl)
                n156 = Less?(x=w373, y=1.6) -> (x < y?=w371:bool)
                n157 = case shown="True" w371 {
                  tunnel: w373 -> [_ w385]
                  frame False {
                    n158 = local read "HTR_Current"() -> (w379:dbl)
                    n159 = Multiply(x=w379, y=1.3) -> (x*y=w378:dbl)
                    n160 = local write "HTR_Current"(w378) -> ()
                  }
                  frame True {
                    n161 = local read "HTR_Current"() -> (w384:dbl)
                    n162 = Multiply(x=w384, y=w385) -> (x*y=w382:dbl)
                    n163 = Less?(x=w382, y=0.00075) -> (x < y?=w381:bool)
                    n164 = case shown="True" w381 {
                      tunnel: w382 -> [_ w387]
                      frame False {
                        n165 = local write "HTR_Current"(0.00075 ("HTR_Current")) -> ()
                      }
                      frame True {
                        n166 = local write "HTR_Current"(w387) -> ()
                      }
                    }
                  }
                }
              }
              frame True {
                n167 = local write "HTR_Current"(w388) -> ()
              }
            }
            n168 = local read "Global Stop"() -> (w363:bool)
          }
          frame "Plot Kxx, Kxy" {
            w406 = Kxx_Kxy_state_machine_cases."End"  # States
            n169 = local read "Sample_Lxx"() -> (w400:dbl)
            n170 = local read "Sample_w"() -> (w402:dbl)
            n171 = local read "Sample_t"() -> (w401:dbl)
            n172 = local read "Sample_Lxy"() -> (w411:dbl)
            n173 = Unbundle By Name(w405) -> ("T_avg"=w404:dbl, "dTxx"=w403:dbl, "dTxy"=w391:dbl, "HTR Power"=w390:dbl)
            n174 = call "Kxx_Kxy_calc.vi"("Sample_w"=w402, "HTR Power"=w390, "Sample_t"=w401, "dTxy"=w391, "dTxx"=w403, "Sample_Lxx"=w400, "Sample_Lxy"=w411) -> ("Kxx"=w410:dbl, "Kxy"=w409:dbl)  [unwired: 3 in]
            n175 = Unbundle By Name(w396) -> ("T_avg data"=w399:dbl[], "Kxx data"=w398:dbl[], "Kxy data"=w397:dbl[])
            n176 = Build Array (concatenate)(w398, w410) -> (w394:dbl[])
            n177 = Build Array (concatenate)(w397, w409) -> (w393:dbl[])
            n178 = Build Array (concatenate)(w399, w404) -> (w395:dbl[])
            n179 = local read "Calibration Only?"() -> (w407:bool)
            n180 = Bundle(w395, w393) -> (w408:cluster{dbl[], dbl[]})  [unwired: 1 in]
            n181 = Bundle(w395, w394) -> (w412:cluster{dbl[], dbl[]})  [unwired: 1 in]
            n182 = Bundle By Name(cluster=w396, "T_avg data"=w395, "Kxx data"=w394, "Kxy data"=w393) -> (w392:T3)
            n183 = case shown="True" w407 {
              tunnel: w412 -> [_ w414]
              tunnel: w408 -> [_ w413]
              frame True {
              }
              frame False {
                "Kxx Plot" <- w414
                "Kxy Plot" <- w413
              }
            }
            n184 = local read "Global Stop"() -> (w389:bool)
          }
          frame "End" {
          }
        }
        n185 = Wait (ms)(milliseconds to wait=u32 10) -> ()  [unwired: 1 out]
      }
      n186 = local read "Global Stop"() -> (w118:bool)
    }
    n187 = local read "Global Stop"() -> (w94:bool)
    "Fieldsp" <- w114
  }
  n188 = Less?(x="Initial Heater Current (A)", y=0.0004) -> (x < y?=w18:bool)
  n189 = case shown="True" w18 {
    tunnel: "Initial Heater Current (A)" -> [_ w420]
    frame False {
      n190 = local write "HTR_Current"(0.0004 ("HTR_Current")) -> ()
    }
    frame True {
      n191 = local write "HTR_Current"(w420) -> ()
    }
  }
  n192 = call <instrlib>:"Initialize.vi"("Reset (True)"=TRUE, "VISA resource name"="DC Voltmeter") -> ("error out"=w74:errorcluster, "VISA resource name out"=w73:refnum<visa-resource-name>)  [unwired: 8 in]
  n193 = VISA Write(VISA resource name=w73, write buffer="INIT:CONT ON", error in (no error)=w74) -> (VISA resource name out=w32:refnum<visa-resource-name>, error out=w31:errorcluster)  [unwired: 1 out]
  n194 = property on="Name" class="Ring (strict)"("Strings []"=w1) -> ()  [unwired: 2 in, 2 out]
  n195 = Tick Count (ms)() -> (millisecond timer value=w23:u32)
  n196 = case shown="True" "Quick Data Recording" {
    tunnel: w22 -> [_ w424]
    tunnel: "Delay (ms)" -> [_ w422]
    tunnel: w1 -> [_ w421]
    frame False {
    }
    frame True {
      # "SAVE DATA TO FILE"
      n197 = Strip Path(path=w424) -> (stripped path=w428:path, name=w425:string)
      n198 = Concatenate Strings(w425, ".dat") -> (w427:string)
      n199 = Tick Count (ms)() -> (millisecond timer value=w431:u32)
      n200 = Build Path(base path=w428, name or relative path=w427) -> (appended path=w429:path)
      n201 = call-poly <vilib>:"Write To Spreadsheet File.vi"("append to file? (new file:F)"=TRUE, "1D data"=w421, "file path (dialog if empty)"=w429) -> ("new file path (Not A Path if cancelled)"=w423:path)  [unwired: 5 in]
      n202 = while {
        tunnel: w431 -> [w456]
        tunnel: w423 -> [w448]
        tunnel: w422 -> [w447]
        stop <- w432 stop-if-true
        n203 = Wait (ms)(milliseconds to wait=w447) -> ()  [unwired: 1 out]
        n204 = Tick Count (ms)() -> (millisecond timer value=w455:u32)
        n205 = global read "MQM Data Transfer All.vi" "ZI MFLI"() -> (w434:T5)
        n206 = Subtract(x=w455, y=w456) -> (x-y=w454:u32)
        n207 = Unbundle By Name(w434) -> ("Lockin 2 Demod 0.X(V)"=w443:dbl, "Lockin 2 Demod 0.Theta (deg)"=w442:dbl)
        n208 = Unbundle By Name(w434) -> ("Lockin 3 Demod 0.X(V)"=w441:dbl, "Lockin 3 Demod 0.Theta (deg)"=w440:dbl)
        n209 = Unbundle By Name(w434) -> ("Lockin 1 Demod 0.X(V)"=w445:dbl, "Lockin 1 Demod 0.Theta (deg)"=w444:dbl)
        n210 = global read "MQM Data Transfer All.vi" "PPMS"() -> (w433:T6)
        n211 = Unbundle By Name(w433) -> ("Temperature.Temperature (K)"=w453:dbl, "Field.Field (T)"=w452:dbl)
        n212 = local read "HTR_Current"() -> (w438:dbl)
        n213 = local read "HTR_Voltage"() -> (w439:dbl)
        n214 = local read "I_therm"() -> (w435:dbl)
        n215 = local read "Mask"() -> (w437:dbl)
        n216 = local read "Tsp"() -> (w436:dbl)
        n217 = Build Array(w454, w453, w452, w445, w444, w443, w442, w441, w440, w439, w438, w437, w436, w435) -> (w451:dbl[])
        n218 = call "Write To Spreadsheet File (DBL)2.vi"("format (%.3f)"="%_8f", "append to file? (new file:F)"=TRUE, "1D data"=w451, "file path (dialog if empty)"=w448) -> ("error out"=w446:errorcluster)  [unwired: 3 in, 1 out]
        n219 = local read "Global Stop"() -> (w432:bool)
        n220 = call <vilib>:"Clear Errors.vi"("error in (no error)"=w446) -> ()  [unwired: 5 in, 2 out]
      }
    }
  }
  n221 = while {
    tunnel: w23 -> [w507]
    shift-right: [w501] -> _
    shift-left: 0 -> [w506]
    tunnel: w1 -> [w502]
    shift-right: [w497] -> _
    shift-left: _ -> [w498]
    tunnel: "Delay (ms)" -> [w491]
    tunnel: w32 -> [w483]
    tunnel: [w463] -> w15
    shift-right: [w462] -> w5
    shift-left: w31 -> [w480]
    stop <- "Finish" stop-if-true
    # "PLOT DATA BEING RECORDED TO FILE CONTINUOUSLY"
    n222 = Wait (ms)(milliseconds to wait=w491) -> ()  [unwired: 1 out]
    n223 = Tick Count (ms)() -> (millisecond timer value=w508:u32)
    n224 = global read "MQM Data Transfer All.vi" "ZI MFLI"() -> (w465:T5)
    n225 = VISA Write(VISA resource name=w483, write buffer="FETC?", error in (no error)=w480) -> (VISA resource name out=w482:refnum<visa-resource-name>, error out=w479:errorcluster)  [unwired: 1 out]
    n226 = Subtract(x=w508, y=w507) -> (x-y=w501:u32)
    n227 = global read "MQM Data Transfer All.vi" "PPMS"() -> (w464:T6)
    n228 = Subtract(x=w501, y=w506) -> (x-y=→"Data Rate (ms)":u32)
    n229 = Unbundle By Name(w465) -> ("Lockin 3 Demod 0.X(V)"=w468:dbl, "Lockin 3 Demod 0.Theta (deg)"=w467:dbl)
    n230 = Unbundle By Name(w465) -> ("Lockin 2 Demod 0.X(V)"=w473:dbl, "Lockin 2 Demod 0.Theta (deg)"=w494:dbl)
    n231 = Unbundle By Name(w464) -> ("Temperature.Temperature (K)"=w500:dbl, "Field.Field (T)"=w499:dbl)
    n232 = Unbundle By Name(w465) -> ("Lockin 1 Demod 0.X(V)"=w471:dbl, "Lockin 1 Demod 0.Theta (deg)"=w470:dbl)
    n233 = VISA Read(VISA resource name=w482, byte count=u32 1000, error in (no error)=w479) -> (VISA resource name out=w463:refnum<visa-resource-name>, read buffer=w478:string, error out=w462:errorcluster)  [unwired: 1 out]
    n234 = Build Array(w501, w500, w499) -> (w495:dbl[])
    n235 = global read "Thermometers.vi" "Thermometers"() -> (w460:cluster{"T_H":dbl, "T_C1":dbl, "T_C2":dbl})
    "Thermometers" <- w460
    n236 = Match Pattern(string=w478, regular expression="VDC", offset (0)=0) -> (before substring=w475:string)  [unwired: 3 out]
    n237 = Build Array (concatenate)(w495, w471, w470) -> (w493:dbl[])
    n238 = local read "HTR_Voltage"() -> (w486:dbl)
    n239 = local read "HTR_Current"() -> (w490:dbl)
    n240 = Fract/Exp String To Number(string=w475) -> (number=w474:dbl)  [unwired: 3 in, 1 out]
    n241 = Build Array (concatenate)(w493, w473, w494) -> (w469:dbl[])
    n242 = local read "I_therm"() -> (w472:dbl)
    n243 = Unbundle By Name(w460) -> ("T_H"=w459:dbl, "T_C1"=w458:dbl, "T_C2"=w457:dbl)
    n244 = local write "HTR_Voltage"(w474) -> ()
    n245 = Build Array (concatenate)(w469, w468, w467) -> (w466:dbl[])
    n246 = local read "Mask"() -> (w488:dbl)
    n247 = local read "Fieldsp"() -> (w461:dbl)
    n248 = local read "Tsp"() -> (w487:dbl)
    n249 = Build Array (concatenate)(w466, w486, w490, w488, w487, w472, w459, w458, w457, w461) -> (w489:dbl[])
    n250 = Build Array (concatenate)(w498, w489) -> (w492:dbl[][])
    n251 = flat-sequence {
      tunnel: "Display Elements" -> [w521]
      tunnel: [w514] -> w505
      tunnel: w502 -> [w510]
      tunnel: w492 -> [w509]
      tunnel: w505 -> [w568]
      frame #0 {
        n252 = for {
          tunnel: w521 -> [w550] mode=indexing
          shift-right: [w542] -> w520
          shift-left: dbl[] [] -> [w541]
          shift-right: [w543] -> w518
          shift-left: dbl[][] [] -> [w552]
          shift-right: [w548] -> w514
          shift-left: string[] [] -> [w547]
          tunnel: w510 -> [w544]
          tunnel: w509 -> [w545]
          i -> [w546]
          n253 = Unbundle By Name(w550) -> ("X"=w551:bool, "Y"=w554:bool, "Name"=w549:u16)
          n254 = Index Array(array=w545, index (col)=w549) -> (element=w553:dbl[])  [unwired: 1 in]
          n255 = case shown="False" w554 {
            tunnel: w553 -> [_ w560]
            tunnel: w552 -> [w558 w567]
            tunnel: [w558 w566] -> w543
            tunnel: w549 -> [_ w565]
            tunnel: [w559 w563] -> w548
            tunnel: w547 -> [w559 w562]
            tunnel: w544 -> [_ w561]
            frame False {
            }
            frame True {
              n256 = Build Array (concatenate)(w567, w560) -> (w566:dbl[][])
              n257 = Index Array(array=w561, index=w565) -> (element=w564:string)
              n258 = Build Array (concatenate)(w562, w564) -> (w563:string[])
            }
          }
          n259 = case shown="False" w551 {
            tunnel: w549 -> [_ w557]
            tunnel: w546 -> [_ _]
            tunnel: w544 -> [_ w555]
            frame False {
            }
            frame True {
              n260 = Index Array(array=w555, index=w557) -> (element=w556:string)
              n261 = property on="All Data" class="XYGraph (strict)"("XScale.NameLbl.Text"=w556) -> ()  [unwired: 2 in, 2 out]
            }
          }
          n262 = Select(t=w553, s=w551, f=w541) -> (s? t:f=w542:dbl[])
        }
        n263 = for {
          tunnel: w518 -> [w525] mode=indexing
          tunnel: w520 -> [w527]
          tunnel: [w528] -> w519 mode=indexing
          n264 = case shown="0, Default" "Y-Axis" {
            tunnel: w525 -> [w529 w531 w534]
            tunnel: [w529 w530 w533] -> w522
            frame 0, Default {
            }
            frame 1 {
              n265 = Reciprocal(x=w531) -> (1/x=w530:dbl[])
            }
            frame 2 {
              n266 = Absolute Value(x=w534) -> (abs(x)=w532:dbl[])
              n267 = Logarithm Base 10(1:w532) -> (0:w533:dbl[])
            }
          }
          n268 = case shown="0, Default" "X-Axis" {
            tunnel: w527 -> [w535 w537 w540]
            tunnel: [w535 w536 w539] -> w526
            frame 0, Default {
            }
            frame 1 {
              n269 = Reciprocal(x=w537) -> (1/x=w536:dbl[])
            }
            frame 2 {
              n270 = Absolute Value(x=w540) -> (abs(x)=w538:dbl[])
              n271 = Logarithm Base 10(1:w538) -> (0:w539:dbl[])
            }
          }
          n272 = Bundle(w526, w522) -> (w528:cluster{dbl[], dbl[]})  [unwired: 1 in]
        }
        "All Data" <- w519
        n273 = Array Size(array=w518) -> (size(s)=w517:i32[])
        n274 = Index Array(array=w517, index=0) -> (element=w515:i32)
        n275 = property on="All Data" class="XYGraph (strict)"("LegNumRows"=w515) -> ()  [unwired: 2 in, 2 out]
      }
      frame #1 {
        n276 = for {
          tunnel: w568 -> [w569] mode=indexing
          i -> [w570]
          n277 = property on="All Data" class="XYGraph (strict)"("Active Plot"=w570, "Plot.Plot Name"=w569) -> ()  [unwired: 2 in, 2 out]
        }
      }
    }
    n278 = call "Data length guard.vi"("Max length"=20000, "Array"=w492) -> ("array w/ subset deleted"=w497:dbl[][])  [unwired: 9 in]
    "Global Stop" <- "Finish"
  }
  n279 = Unbundle By Name(w14) -> ("error out"=w13:errorcluster)
  n280 = call <instrlib>:"SetTemperature.vi"("Rate"=3.0, "Temperature"="Final Temperature (K)", "error in (no error)"=w13, "Instrument Ref In"=w11) -> ("error out"=w28:errorcluster, "Instrument Ref Out"=w29:refnum<k24>)  [unwired: 3 in, 1 out]
  n281 = call <instrlib>:"SetField.vi"("Rate"=100.0, "Field"="Final Field (Oe)", "error in (no error)"=w28, "Instrument Ref In"=w29) -> ("error out"=→"QD error out":errorcluster)  [unwired: 3 in, 2 out]
  n282 = VISA Close(VISA resource name=w3) -> ()  [unwired: 1 in, 1 out]
  n283 = VISA Close(VISA resource name=w10, error in (no error)=w7) -> (error out=→"KE6221 error out":errorcluster)
  n284 = VISA Close(VISA resource name=w15, error in (no error)=w5) -> (error out=→"KE2182 error out":errorcluster)
